vi "Resp LPF.vi"(6 "Filter Order":i32=8, 7 "Enable":bool, 8 "error in (no error)":errorcluster, 9 "Cutoff Frequency":dbl=2.0 format="%0.4fHz", 10 "Data Rate":dbl=500.0 format="%^#_6gSPS", 11 "Data In":dbl[](array[numeric])) -> (0 "error out":errorcluster, 3 "Filtered Data":dbl[](array[numeric]))   [LabVIEW 2010]
doc: "This VI applies a low-pass filter to the input data array (Respiration Data).\n\nInputs:\nEnable - (bool) TRUE = enable the filter, FALSE = do not filter (data is passed through)\nData In - (DBL[]) respiration data array to filter\nData Rate - (DBL) data rate of Data In (SPS)\nCutoff Frequency - (DBL) low-pass filter cutoff frequency (Hz)\nFilter Order - (I32) order of low-pass filter\nerror in - error input cluster\n\nOutputs:\nFiltered Data - (DBL[]) respiration data after filter is applied (or pass through for filter not enabled)\nerror out - error output cluster"
uses:
  <vilib>/Analysis/3filter.llb/Butterworth Filter (DBL).vi
  <vilib>/Analysis/NI_AALBase.lvlib
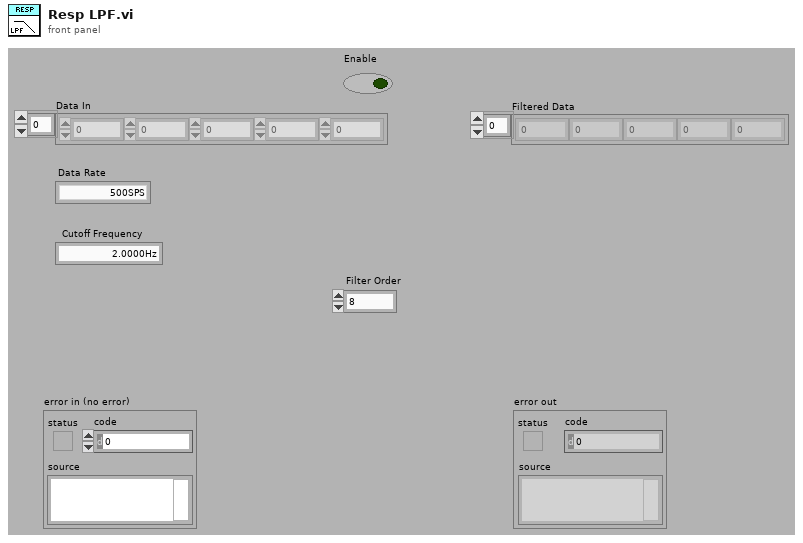
[diagram p1: front panel]
types:
  T1 = enum32{"Lowpass", "Highpass", "Bandpass", "Bandstop"}
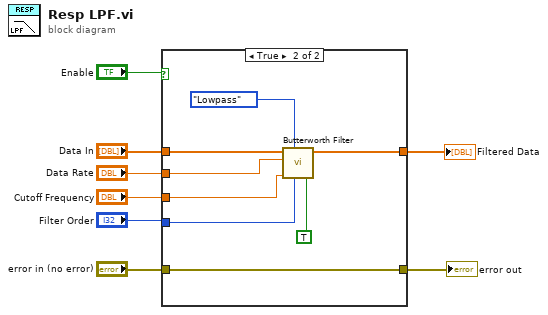
[diagram p0: block diagram]
diagram:
  n1 = case shown="True" "Enable" {
    tunnel: "error in (no error)" -> [w10 w16]
    tunnel: [w10 w16] -> w6
    tunnel: [w9 w15] -> w5
    tunnel: "Data In" -> [w9 w14]
    tunnel: "Data Rate" -> [_ w13]
    tunnel: "Cutoff Frequency" -> [_ w12]
    tunnel: "Filter Order" -> [_ w11]
    frame False {
    }
    frame True {
      n2 = call-poly <vilib>:"Butterworth Filter.vi"("init/cont (init:F)"=TRUE, "order"=w11, "filter type"=T1."Lowpass", "low cutoff freq: fl"=w12, "sampling freq: fs"=w13, "X"=w14) -> ("Filtered X"=w15:dbl[])  [unwired: 1 in, 2 out]
    }
  }
  "Filtered Data" <- w5
  "error out" <- w6
